vi "Stop Core.vi"(10 "final error code":i32, 11 "[V] Login in":refnum<class "[V] Login.lvclass">) -> (3 "[V] Login out":refnum<class "[V] Login.lvclass">)   [LabVIEW 2020, in "[V] Login.lvlib" / "[V] Login.lvclass"]
doc: "(<B>Filename</B>: Actor Framework.lvlib:Actor.lvclass:Stop Core.vi)\n\nDefines what the actor does before it stops. Use the <B>final error code</B> input to determine whether the actor shut down in response to an error.\n\nBy default, this method passes the Stop message along to all auto-stop nested actors. A descendant class may override this method to define additional behavior, such as shutting down any processes the actor initiated in its override of the Actor Core method."
uses:
  [V] Login.lvclass
  [V] Login.lvclass/[V] Login.ctl
  <vilib>/ActorFramework/Actor/Actor.lvclass
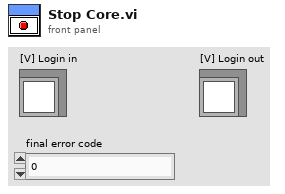
[diagram p1: front panel]
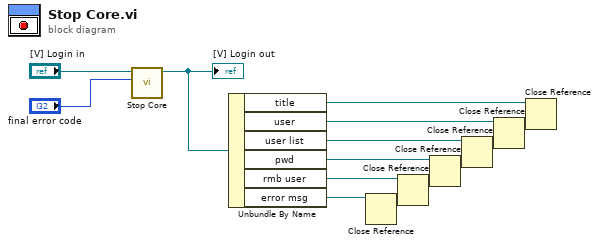
[diagram p0: block diagram]
diagram:
  n1 = call-parent "Stop Core.vi"("final error code"="final error code", "Actor in"="[V] Login in") -> ("Actor out"=w7:refnum<class "[V] Login.lvclass">)  [unwired: 9 in]
  "[V] Login out" <- w7
  n2 = Unbundle By Name(w7) -> ("title"=w6:refnum<vi>, "user"=w5:refnum<vi>, "user list"=w4:refnum<vi>, "pwd"=w3:refnum<vi>, "rmb user"=w2:refnum<vi>, "error msg"=w1:refnum<vi>)
  n3 = Close Reference(reference=w1) -> ()  [unwired: 1 in, 1 out]
  n4 = Close Reference(reference=w2) -> ()  [unwired: 1 in, 1 out]
  n5 = Close Reference(reference=w3) -> ()  [unwired: 1 in, 1 out]
  n6 = Close Reference(reference=w4) -> ()  [unwired: 1 in, 1 out]
  n7 = Close Reference(reference=w5) -> ()  [unwired: 1 in, 1 out]
  n8 = Close Reference(reference=w6) -> ()  [unwired: 1 in, 1 out]
